vi "SetDragInfo__slk_mt.vi"(8 "error in (no error)":errorcluster, 11 "tree view in":refnum<class "TreeView__slk_mt.lvclass">) -> (0 "error out":errorcluster, 3 "tree view out":refnum<class "TreeView__slk_mt.lvclass">)   [LabVIEW 2013, in "Lazyboots Menu Tool.lvlib" / "TreeView__slk_mt.lvclass"]
doc: "Sets drag information."
uses:
  TreeView__slk_mt.lvclass
panel:
  # "SetDragInfo__slk_mt.vi\nSets drag information.\n\nNOTICE -- YOU MUST LEAVE THIS NOTICE IN PLACE.\n\nCopyright (c) 2011, LIANG LIU Shawn.Liu.cn@gmail.com\nAll rights reserved.\n\nRedistribution and use in source and binary forms, with or without modification, are permitted provided that the following conditions are met:\n-Redistributions of source code must retain the above copyright notice, this list of conditions and the following disclaimer.\n-Redistributions in binary form must reproduce the above copyright notice, this list of conditions and the following disclaimer in the documentation and/or other materials provided with the distribution.\n-Neither the name of the eLp nor the names of its contributors may be used to endorse or promote products derived from this software without specific prior written permission.\n\nTHIS SOFTWARE IS PROVIDED BY THE COPYRIGHT HOLDERS AND CONTRIBUTORS \"AS IS\" AND ANY EXPRESS OR IMPLIED WARRANTIES, INCLUDING, BUT NOT LIMITED TO, THE IMPLIED WARRANTIES OF MERCHANTABILITY AND FITNESS FOR A PARTICULAR PURPOSE ARE DISCLAIMED. IN NO EVENT SHALL THE COPYRIGHT HOLDER OR CONTRIBUTORS BE LIABLE FOR ANY DIRECT, INDIRECT, INCIDENTAL, SPECIAL, EXEMPLARY, OR CONSEQUENTIAL DAMAGES (INCLUDING, BUT NOT LIMITED TO, PROCUREMENT OF SUBSTITUTE GOODS OR SERVICES; LOSS OF USE, DATA, OR PROFITS; OR BUSINESS INTERRUPTION) HOWEVER CAUSED AND ON ANY THEORY OF LIABILITY, WHETHER IN CONTRACT, STRICT LIABILITY, OR TORT (INCLUDING NEGLIGENCE OR OTHERWISE) ARISING IN ANY WAY OUT OF THE USE OF THIS SOFTWARE, EVEN IF ADVISED OF THE POSSIBILITY OF SUCH DAMAGE."
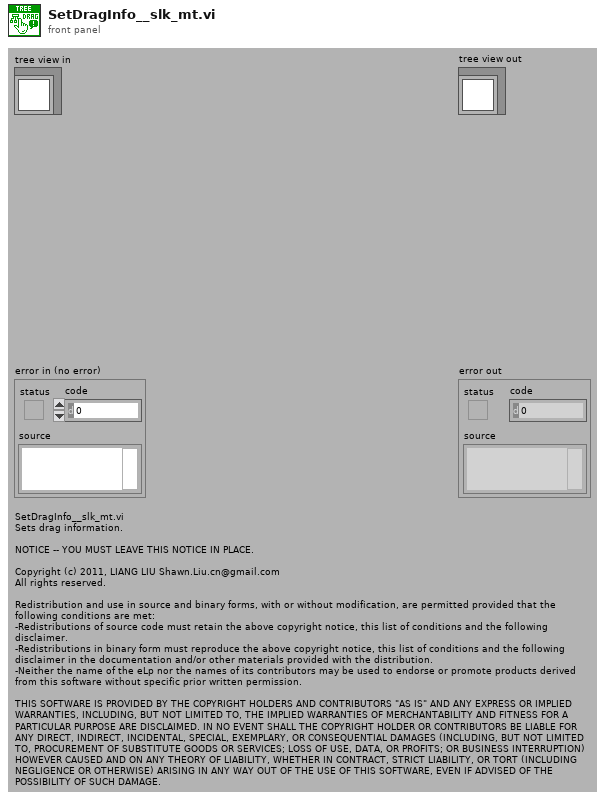
[diagram p1: front panel]
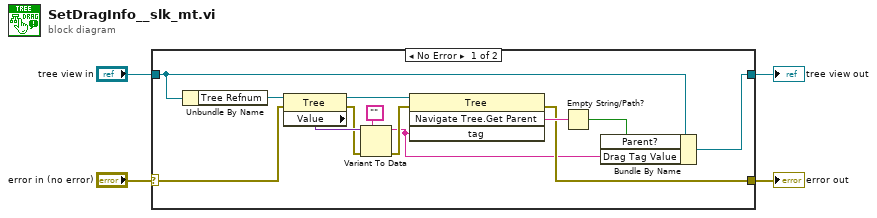
[diagram p0: block diagram]
diagram:
  n1 = case shown="No Error" "error in (no error)" {
    selector: "error in (no error)" -> [w8 w19]
    tunnel: [w12 w19] -> w3
    tunnel: [w13 w18] -> w1
    tunnel: "tree view in" -> [w14 w18]
    frame No Error {
      n2 = Unbundle By Name(w14) -> ("Tree Refnum"=w17:refnum<vi>)
      n3 = property class="Tree"(reference=w17, error in=w8) -> (reference out=w11:refnum<vi>, error out=w7:errorcluster, "Value"=w10:variant)
      n4 = Variant To Data(error in=w7, type="", Variant=w10) -> (data=w5:string, error out=w6:errorcluster)
      n5 = invoke class="Tree" method="Navigate Tree.Get Parent"(reference=w11, error in=w6, "tag"=w5) -> (error out=w12:errorcluster, "Navigate Tree:Get Parent"=w15:string)  [unwired: 1 in, 2 out]
      n6 = Empty String/Path?(string/path=w15) -> (empty?=w16:bool)
      n7 = Bundle By Name(cluster=w14, "Parent?"=w16, "Drag Tag Value"=w5) -> (w13:refnum<class "TreeView__slk_mt.lvclass">)
    }
    frame Error {
    }
  }
  "error out" <- w3
  "tree view out" <- w1
